vi "XIPIN_FIR_Compiler_5_0.vi"   [LabVIEW 2017]
doc: "The Xilinx FIR Compiler LogiCORE is a module for generation of high speed, compact filter implementations that can be configured to implement many different filtering functions. The core is fully synchronous, using a single clock, and is highly parameterizable, allowing designers to control the filter type, data and coefficient widths, the number of filter taps, the number of channels, etc. Multi-rate operation is supported. The implementation method can be specified by the user, with a choice of Multiply-Accumulate or Distributed Arithmetic architectures. The core is delivered through the Xilinx CORE Generator System and integrates seamlessly with the Xilinx design flow.\n------------------------------------\n<b>Need License</b> : No"
uses:
  <vilib>/rvi/XilinxIP/XIPIN_XNode/niFpgaXIPIN.xnode
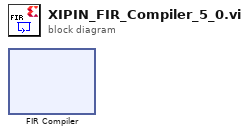
[diagram p0: block diagram]
diagram:
  n1 = xnode ("FIR Compiler")() -> ()
